vi "Update AbsoluteResolution.vi"(8 "error in (no error)":errorcluster, 10 "absolute resolution (0.001)":dbl=0.001 format="%^.2e", 11 "CS++DMMGui in":refnum<class "CS++DMMGui.lvclass">) -> (0 "error out":errorcluster, 3 "CS++DMMGui out":refnum<class "CS++DMMGui.lvclass">)   [LabVIEW 2013, in "CS++DMMGui.lvlib" / "CS++DMMGui.lvclass"]
doc: "Update value of absolute resolution on GUI via event."
uses:
  CS++DMMGui.lvclass
  CS++DMMGui.lvclass/CS++DMMGui.ctl
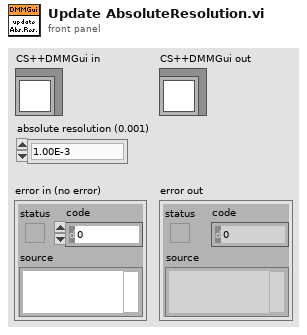
[diagram p1: front panel]
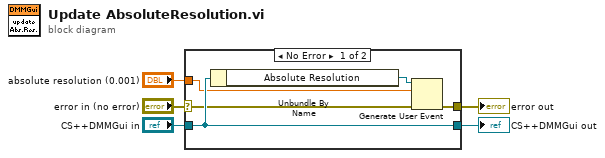
[diagram p0: block diagram]
diagram:
  n1 = case shown="No Error" "error in (no error)" {
    selector: "error in (no error)" -> [w7 w12]
    tunnel: [w6 w12] -> w4
    tunnel: [w10 w11] -> w2
    tunnel: "CS++DMMGui in" -> [w10 w11]
    tunnel: "absolute resolution (0.001)" -> [w8 _]
    frame No Error {
      n2 = Unbundle By Name(w10) -> ("Absolute Resolution"=w9:refnum<user-event>)
      n3 = Generate User Event(user event=w9, event data cluster=w8, error in=w7) -> (error out=w6:errorcluster)  [unwired: 1 in, 1 out]
    }
    frame Error {
    }
  }
  "error out" <- w4
  "CS++DMMGui out" <- w2
